vi "2020-ShooterMotor.vi"(8 "error in":errorcluster, 11 "Boolean":bool) -> (0 "error out":errorcluster)   [LabVIEW 2020]
uses:
  2020LabView/2020-Robot Global Data.vi
  <vilib>/Rock Robotics/WPI/ThirdParty/Phoenix-LabVIEW/Motor Controller/Controls/CTRE_Phoenix_MotorControl_ControlMode.ctl
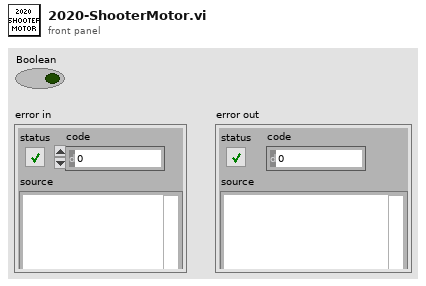
[diagram p1: front panel]
types:
  T1 = typedef "CTRE_Phoenix_MotorControl_ControlMode.ctl" = u16
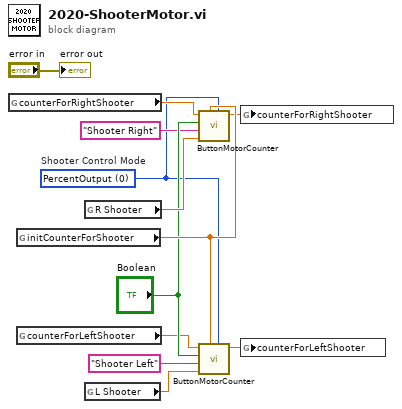
[diagram p0: block diagram]
diagram:
  w1 = T1 0 items=["PercentOutput"=0, "Position"=1, "Velocity"=2, "Current"=3, "Follower"=5, "MotionProfile"=6, "MotionMagic"=7, "MotionProfileArc"=10, "Disabled"=15]  # Shooter Control Mode
  n1 = global read "2020-Robot Global Data.vi" "counterForRightShooter"() -> (w8:dbl)
  n2 = global read "2020-Robot Global Data.vi" "initCounterForShooter"() -> (w12:dbl)
  n3 = global read "2020-Robot Global Data.vi" "counterForLeftShooter"() -> (w5:dbl)
  n4 = global read "2020-Robot Global Data.vi" "R Shooter"() -> (w10:dbl)
  n5 = global read "2020-Robot Global Data.vi" "L Shooter"() -> (w11:dbl)
  n6 = call "ButtonMotorCounter.vi"("Motor Controller Control Mode"=w1, "counterStartValue"=w12, "Motor Set Point"=w10, "refnum name"="Shooter Right", "Boolean"="Boolean", "counterForIntake in"=w8) -> ("counterForIntake out"=w6:dbl)  [unwired: 4 in, 1 out]
  n7 = call "ButtonMotorCounter.vi"("Motor Controller Control Mode"=w1, "counterStartValue"=w12, "Motor Set Point"=w11, "refnum name"="Shooter Left", "Boolean"="Boolean", "counterForIntake in"=w5) -> ("counterForIntake out"=w3:dbl)  [unwired: 4 in, 1 out]
  n8 = global write "2020-Robot Global Data.vi" "counterForRightShooter"(w6) -> ()
  n9 = global write "2020-Robot Global Data.vi" "counterForLeftShooter"(w3) -> ()
  "error out" <- "error in"
